vi "Wrist SetPoint Sequencer.vi"(10 "dt":u32=1500, 11 "SetPoint":dbl format="%#_13g") -> (3 "Active SetPoint":dbl)   [LabVIEW 2018]
uses:
  <vilib>/ptbypt/NI_PtbyPt.lvlib
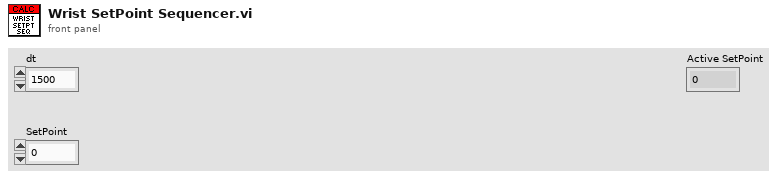
[diagram p1: front panel]
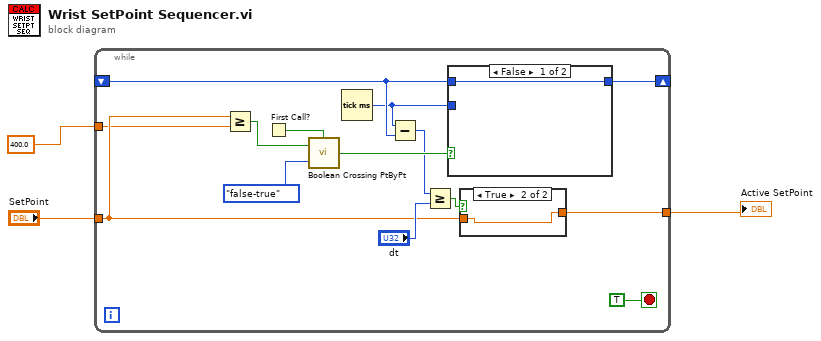
[diagram p0: block diagram]
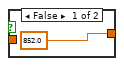
[diagram p2: hidden frame]
diagram:
  n1 = while {
    shift-right: [w16] -> _
    shift-left: _ -> [w12]
    tunnel: "SetPoint" -> [w8]
    tunnel: 400.0 ("threshold") -> [w7]
    tunnel: [w6] -> w1
    stop <- TRUE stop-if-true
    n2 = Greater Or Equal?(x=w8, y=w7) -> (x >= y?=w15:bool)
    n3 = First Call?() -> (First Call?: T/F=w5:bool)
    n4 = call <vilib>:"Boolean Crossing PtByPt.vi"("initialize"=w5, "direction"=enum16{"either", "false-true", "true-false"}."false-true", "input"=w15) -> ("crossing"=w13:bool)
    n5 = Tick Count (ms)() -> (millisecond timer value=w4:u32)
    n6 = Subtract(x=w4, y=w12) -> (x-y=w11:u32)
    n7 = Greater Or Equal?(x=w11, y="dt") -> (x >= y?=w9:bool)
    n8 = case shown="False" w13 {
      tunnel: [w20 w21] -> w16
      tunnel: w12 -> [w20 _]
      tunnel: w4 -> [_ w21]
      frame False {
      }
      frame True {
      }
    }
    n9 = case shown="True" w9 {
      tunnel: [852.0 ("max setpt") w19] -> w6
      tunnel: w8 -> [_ w19]
      frame False {
      }
      frame True {
      }
    }
  }
  "Active SetPoint" <- w1
